vi "Send Remove a Dev Requested by UI.vi"(8 "error in (no error)":errorcluster, 10 "DevInfo":refnum<class "DevInfo.lvclass">, 11 "Message Enqueuer in":refnum<class "Message Enqueuer.lvclass">) -> (0 "error out":errorcluster, 3 "Message Enqueuer out":refnum<class "Message Enqueuer.lvclass">)   [LabVIEW 2016, in "Controller Actor.lvlib" / "Remove a Dev Requested by UI Msg.lvclass"]
uses:
  <userlib>/Common Components/Controller/Messages/Remove a Dev Requested by UI Msg/Remove a Dev Requested by UI Msg.lvclass
  <userlib>/Common Components/Hardware/DevInfo/DevInfo.lvclass
  <vilib>/ActorFramework/Message Enqueuer/Message Enqueuer.lvclass
  C:/Program Files (x86)/National Instruments/LabVIEW 2016/vi.lib/ActorFramework/Message/Message.lvclass
  <userlib>/Common Components/Controller/Messages/Remove a Dev Requested by UI Msg/Remove a Dev Requested by UI Msg.lvclass/Remove a Dev Requested by UI Msg.ctl
  <vilib>/ActorFramework/Message Enqueuer/Message Enqueuer.lvclass/Message Enqueuer.ctl
  <vilib>/ActorFramework/Message Priority Queue/Priority Enqueue.vi
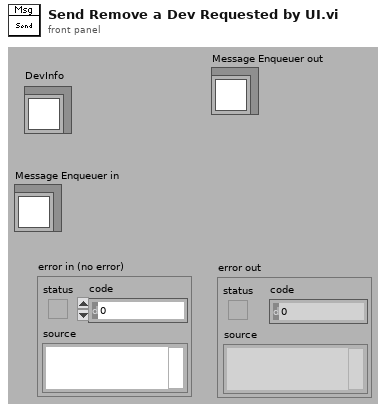
[diagram p1: front panel]
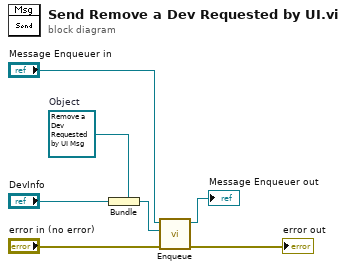
[diagram p0: block diagram]
diagram:
  w7 = refnum<class "Remove a Dev Requested by UI Msg.lvclass"> refnum  # Object
  n1 = Bundle(cluster=w7, "DevInfo") -> (w5:refnum<class "Remove a Dev Requested by UI Msg.lvclass">)
  n2 = call <vilib>:"Enqueue.vi"("error in (no error)"="error in (no error)", "Message"=w5, "Message Enqueuer in"="Message Enqueuer in") -> ("error out"=→"error out":errorcluster, "Message Enqueuer out"=→"Message Enqueuer out":refnum<class "Message Enqueuer.lvclass">)  [unwired: 7 in]
